vi "LEIN m serial Interface settings.vi"(0 "baud rate":u32=9600, 1 "Action(GET)":enum16{"GET", "SET"}(ring), 5 "Reply timeout":u32=700, 7 "LEIN m serial VISA  name  in":refnum<visa-resource-name>, 9 "Modem sim in":T1={"Modem dealay sim"=FALSE, "Sim baud Tx"=1200, "Bit Error fraction Tx"=0.0, "Sim baud Rx"=1200, "Bit Error fraction Rx"=0.0} {"Bit Error fraction Rx" format="%.9f"; "Sim baud Rx" items=["9600"=9600, "4800"=4800, "2400"=2400, "1200"=1200, "1000"=1000, "800"=800, "600"=600, "400"=400, "200"=200]; "Bit Error fraction Tx" format="%.9f"; "Sim baud Tx" items=["9600"=9600, "4800"=4800, "2400"=2400, "1200"=1200, "1000"=1000, "800"=800, "600"=600, "400"=400, "200"=200]}, 11 "error in (no error)":errorcluster) -> (4 "baud rate out":u32, 6 "Timeout out":u32, 8 "LEIN m  Visa name  out":refnum<visa-resource-name>, 10 "Modem sim out":T1={"Modem dealay sim"=FALSE, "Sim baud Tx"=1200, "Bit Error fraction Tx"=0.0, "Sim baud Rx"=1200, "Bit Error fraction Rx"=0.0} {"Bit Error fraction Rx" format="%.9f"; "Sim baud Rx" items=["9600"=9600, "4800"=4800, "2400"=2400, "1200"=1200, "1000"=1000, "800"=800, "600"=600, "400"=400, "200"=200]; "Bit Error fraction Tx" format="%.9f"; "Sim baud Tx" items=["9600"=9600, "4800"=4800, "2400"=2400, "1200"=1200, "1000"=1000, "800"=800, "600"=600, "400"=400, "200"=200]}, 14 "Changed since last get":bool, 15 "error out":errorcluster)   [LabVIEW 2011]
uses:
  GUI/Options/Modem simulation setup.ctl
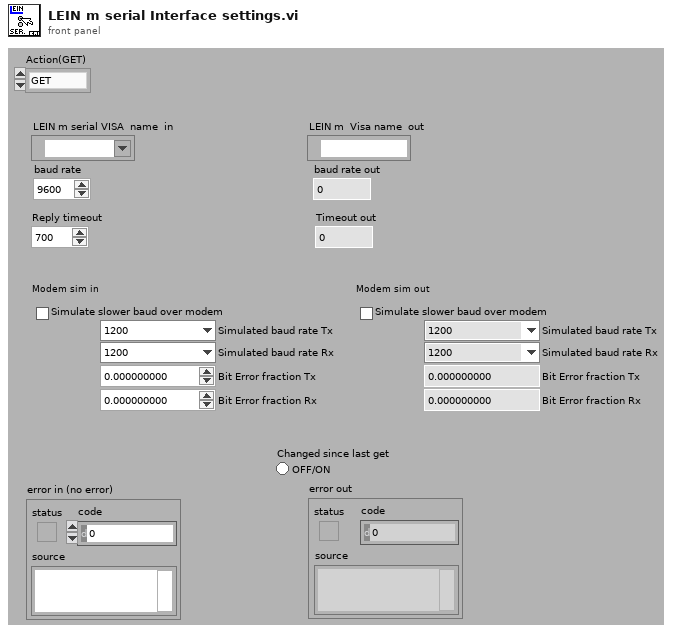
[diagram p1: front panel]
types:
  T1 = typedef "Modem simulation setup.ctl" = cluster{"Modem dealay sim":bool, "Sim baud Tx":u16, "Bit Error fraction Tx":dbl, "Sim baud Rx":u16, "Bit Error fraction Rx":dbl}
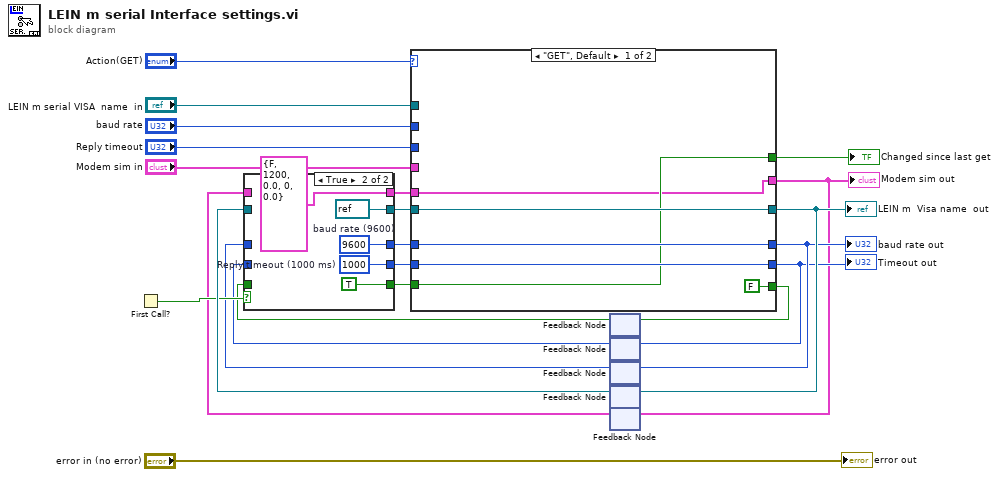
[diagram p0: block diagram]
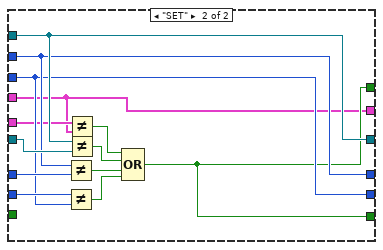
[diagram p3: hidden frame]
diagram:
  n1 = First Call?() -> (First Call?: T/F=w20:bool)
  n2 = feedback #1() -> (w8:bool)  [unwired: 1 in]
  n3 = feedback #2() -> (w12:u32)  [unwired: 1 in]
  n4 = feedback #3() -> (w13:u32)  [unwired: 1 in]
  n5 = feedback #4() -> (w21:refnum<visa-resource-name>)  [unwired: 1 in]
  n6 = feedback #5() -> (w2:T1)  [unwired: 1 in]
  n7 = case shown="True" w20 {
    tunnel: w21 -> [w28 _]
    tunnel: [w28 refnum<visa-resource-name> refnum ("PCP VISA  name")] -> w18
    tunnel: [w27 w32] -> w15
    tunnel: [w26 w31] -> w14
    tunnel: w13 -> [w27 _]
    tunnel: w12 -> [w26 _]
    tunnel: w8 -> [w25 _]
    tunnel: [w25 TRUE] -> w7
    tunnel: w2 -> [w24 _]
    tunnel: [w24 T1 {"Modem dealay sim"=FALSE, "Sim baud Tx"=1200, "Bit Error fraction Tx"=0.0, "Sim baud Rx"=0, "Bit Error fraction Rx"=0.0} ("Modem sim in")] -> w1
    frame False {
    }
    frame True {
      w31 = u32 1000  # Reply timeout (1000 ms)
      w32 = u32 9600  # baud rate (9600)
    }
  }
  n8 = case shown="\"GET\", Default" "Action(GET)" {
    tunnel: [w39 w51] -> w19
    tunnel: w18 -> [w39 w52]
    tunnel: "LEIN m serial VISA  name  in" -> [_ w51]
    tunnel: [w38 w48] -> w16
    tunnel: w15 -> [w38 w50]
    tunnel: [w37 w47] -> w5
    tunnel: w14 -> [w37 w49]
    tunnel: "baud rate" -> [_ w48]
    tunnel: "Reply timeout" -> [_ w47]
    tunnel: [FALSE w43] -> w9
    tunnel: w7 -> [w35 _]
    tunnel: [w35 w43] -> w6
    tunnel: "Modem sim in" -> [_ w41]
    tunnel: [w34 w41] -> w3
    tunnel: w1 -> [w34 w42]
    frame "GET", Default {
    }
    frame "SET" {
      n9 = Not Equal?(x=w48, y=w50) -> (x != y?=w45:bool)
      n10 = Not Equal?(x=w49, y=w47) -> (x != y?=w44:bool)
      n11 = Not Equal?(x=w42, y=w41) -> (x != y?=w40:bool)
      n12 = Not Equal?(x=w51, y=w52) -> (x != y?=w46:bool)
      n13 = Compound Arithmetic op=OR(w40, w46, w45, w44) -> (w43:bool)
    }
  }
  "LEIN m  Visa name  out" <- w19
  "Changed since last get" <- w6
  "baud rate out" <- w16
  "Timeout out" <- w5
  "Modem sim out" <- w3
  n14 = feedback-in #1(w9) -> ()
  n15 = feedback-in #2(w5) -> ()
  n16 = feedback-in #3(w16) -> ()
  n17 = feedback-in #4(w19) -> ()
  n18 = feedback-in #5(w3) -> ()
  "error out" <- "error in (no error)"
